vi "Read Message.vi"(8 "error in (no error)":errorcluster, 11 "RemoteControl in":refnum<class "RemoteControl.lvclass">) -> (0 "error out":errorcluster, 2 "Message":T1, 3 "RemoteControl out":refnum<class "RemoteControl.lvclass">)   [LabVIEW 2019, in "RemoteControl.lvlib" / "RemoteControl.lvclass"]
uses:
  RemoteControl.lvclass
  Typedefs/Message--Cluster.ctl
  RemoteControl.lvclass/RemoteControl.ctl
  Private/RemoteControl.GlobalVariable.vi
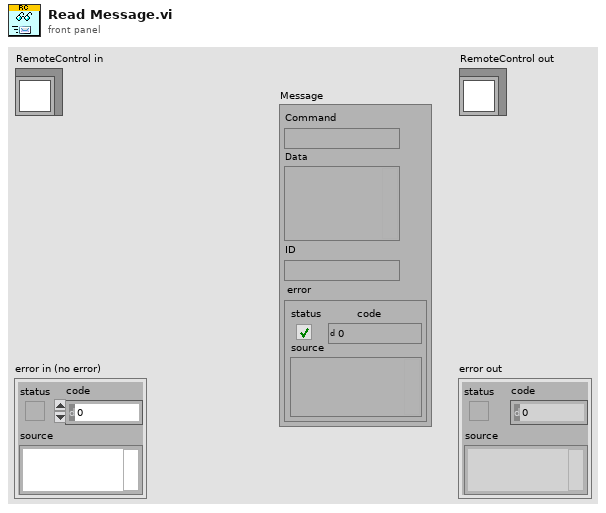
[diagram p1: front panel]
types:
  T1 = typedef "RemoteControl.lvlib/RemoteControl.lvclass/Message--Cluster.ctl" = cluster{"Command":string, "Data":variant, "ID":string, "error":errorcluster}
  T2 = typedef "RemoteControl.lvlib/RemoteControl.lvclass/RC Process Type--Enum.ctl" = enum16{"Listener", "Server", "Client"}
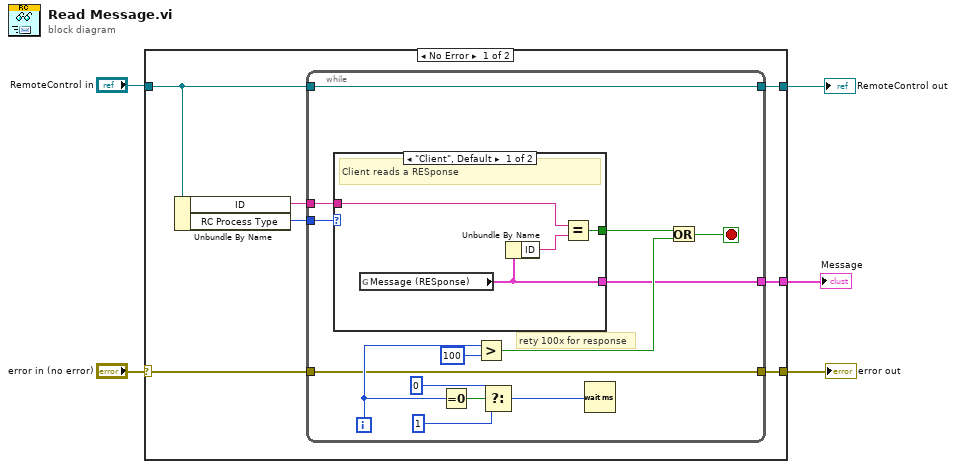
[diagram p0: block diagram]
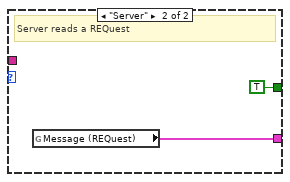
[diagram p2: hidden frame]
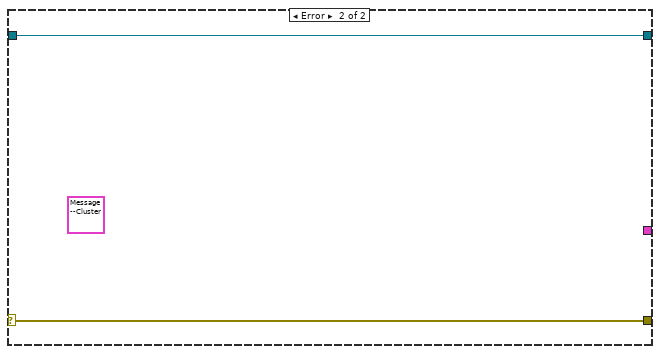
[diagram p3: hidden frame]
diagram:
  n1 = case shown="No Error" "error in (no error)" {
    selector: "error in (no error)" -> [w12 w33]
    tunnel: [w8 w34] -> w3
    tunnel: "RemoteControl in" -> [w7 w34]
    tunnel: [w11 w33] -> w2
    tunnel: [w6 _] -> w1
    frame No Error {
      n2 = Unbundle By Name(w7) -> ("ID"=w9:string, "RC Process Type"=w10:T2)
      n3 = while {
        tunnel: w10 -> [w26]
        tunnel: w9 -> [w25]
        tunnel: w12 -> [w13]
        tunnel: [w13] -> w11
        tunnel: w7 -> [w15]
        tunnel: [w15] -> w8
        tunnel: [w14] -> w6
        i -> [w20]
        stop <- w17 stop-if-true
        # "rety 100x for response"
        n4 = case shown="\"Client\", Default" w26 {
          tunnel: [w30 w32] -> w14
          tunnel: w25 -> [w27 _]
          tunnel: [w29 TRUE] -> w18
          frame "Client", Default {
            # "Client reads a RESponse"
            n5 = global read "RemoteControl.GlobalVariable.vi" "Message (RESponse)"() -> (w30:T1)
            n6 = Unbundle By Name(w30) -> ("ID"=w28:string)
            n7 = Equal?(x=w27, y=w28) -> (x = y?=w29:bool)
          }
          frame "Server" {
            # "Server reads a REQuest"
            n8 = global read "RemoteControl.GlobalVariable.vi" "Message (REQuest)"() -> (w32:T1)
          }
        }
        n9 = Equal To 0?(x=w20) -> (x = 0?=w24:bool)
        n10 = Greater?(x=w20, y=100) -> (0:w16:bool)
        n11 = Select(t=u32 0 ("milliseconds to wait"), s=w24, f=u32 1 ("milliseconds to wait")) -> (s? t:f=w21:u32)
        n12 = Wait (ms)(milliseconds to wait=w21) -> ()  [unwired: 1 out]
        n13 = Or(x=w18, y=w16) -> (x .or. y?=w17:bool)
      }
    }
    frame Error {
      (unwired) T1 {"Command"="", "Data"=variant(string ""), "ID"="", "error"={"status"=FALSE, "code"=0, "source"=""}} ("Message")
    }
  }
  "error out" <- w2
  "RemoteControl out" <- w3
  "Message" <- w1
